vi "Configure Modulation (Frequency).vi"(0 "VISA resource name":refnum<visa-resource-name>, 1 "Enable Frequency Modulation (T: Enable)":bool=TRUE, 5 "Channel (0: Channel 1)":u16(ring) items=["Channel 1", "Channel 2"], 7 "FM Source (0: Internal)":u16(ring) items=["Internal", "External"], 9 "Modulation Waveform (0: Sine)":u16(ring) items=["Sine", "Square", "Triangle", "Ramp", "Down Ramp", "Noise", "User 1", "User 2", "User 3", "User 4", "Edit Memory"], 11 "error in (no error)":errorcluster, 12 "Modulation Frequency (100.00 Hz)":dbl=100.0, 13 "Peak Deviation (100.00 Hz)":dbl=100.0) -> (4 "VISA resource name out":refnum<visa-resource-name>, 15 "error out":errorcluster)   [LabVIEW 2020, in "AWG.lvlib" / "Tektronix AFG 3000 Series.lvlib"]
doc: "Configures and enables frequency modulation (FM). In FM, the frequency of the carrier is varied by the frequency of the modulating waveform."
uses:
  Tektronix AFG 3000 Series.lvlib
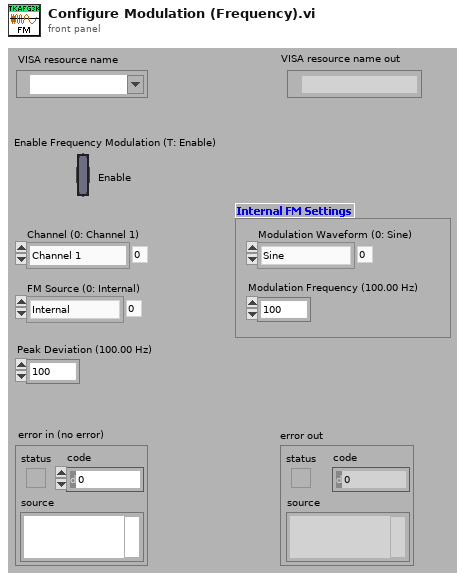
[diagram p1: front panel]
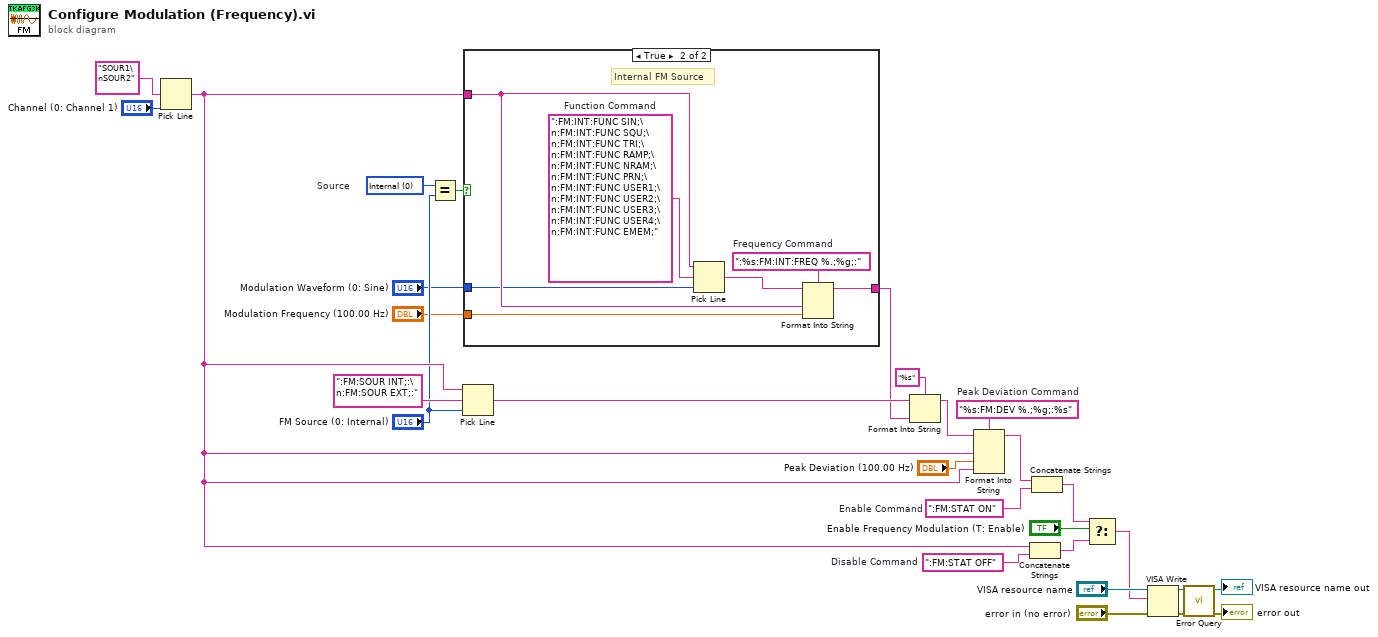
[diagram p0: block diagram]
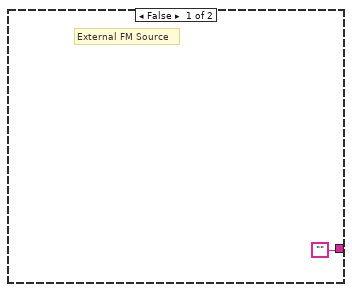
[diagram p2: hidden frame]
diagram:
  w19 = ":FM:STAT ON"  # Enable Command
  w7 = u16 0 items=["Internal", "External"]  # Source
  w22 = "%s:FM:DEV %.;%g;:%s"  # Peak Deviation Command
  w16 = ":FM:STAT OFF"  # Disable Command
  n1 = Pick Line(multi-line string="SOUR1\nSOUR2" ("string (\"\")"), line index="Channel (0: Channel 1)") -> (output string=w10:string)  [unwired: 1 in]
  n2 = Equal?(x=w7, y="FM Source (0: Internal)") -> (x = y?=w9:bool)
  n3 = Pick Line(string ("")=w10, multi-line string=":FM:SOUR INT;:\n:FM:SOUR EXT;:" ("Source Command"), line index="FM Source (0: Internal)") -> (output string=w5:string)
  n4 = case shown="True" w9 {
    tunnel: ["" w33] -> w4
    tunnel: w10 -> [_ w32]
    tunnel: "Modulation Waveform (0: Sine)" -> [_ w31]
    tunnel: "Modulation Frequency (100.00 Hz)" -> [_ w30]
    frame False {
      # "External FM Source"
    }
    frame True {
      w34 = ":FM:INT:FUNC SIN;\n:FM:INT:FUNC SQU;\n:FM:INT:FUNC TRI;\n:FM:INT:FUNC RAMP;\n:FM:INT:FUNC NRAM;\n:FM:INT:FUNC PRN;\n:FM:INT:FUNC USER1;\n:FM:INT:FUNC USER2;\n:FM:INT:FUNC USER3;\n:FM:INT:FUNC USER4;\n:FM:INT:FUNC EMEM;"  # Function Command
      w36 = ":%s:FM:INT:FREQ %.;%g;:"  # Frequency Command
      # "Internal FM Source"
      n5 = Pick Line(string ("")=w32, multi-line string=w34, line index=w31) -> (output string=w35:string)
      n6 = Format Into String(format string=w36, initial string=w35, w32, w30) -> (resulting string=w33:string)  [unwired: 1 in, 1 out]
    }
  }
  n7 = Format Into String(format string="%s", initial string=w5, w4) -> (resulting string=w3:string)  [unwired: 1 in, 1 out]
  n8 = Format Into String(format string=w22, initial string=w3, w10, "Peak Deviation (100.00 Hz)", w10) -> (resulting string=w20:string)  [unwired: 1 in, 1 out]
  n9 = Concatenate Strings(w10, w16) -> (w14:string)
  n10 = Concatenate Strings(w20, w19) -> (w12:string)
  n11 = Select(t=w12, s="Enable Frequency Modulation (T: Enable)", f=w14) -> (s? t:f=w13:string)
  n12 = VISA Write(VISA resource name="VISA resource name", write buffer=w13, error in (no error)="error in (no error)") -> (VISA resource name out=w25:refnum<visa-resource-name>, error out=w26:errorcluster)  [unwired: 1 out]
  n13 = call "Error Query.vi"("error in (no error)"=w26, "VISA resource name"=w25) -> ("error out"=→"error out":errorcluster, "VISA resource name out"=→"VISA resource name out":refnum<visa-resource-name>)  [unwired: 6 in, 2 out]
